vi "Get Session Info - 1Pin MSess .vi"(8 "error in":errorcluster, 10 "pin or relay name":string, 11 "session reservation in":refnum<class "Session Reservation.lvclass">) -> (0 "error out":errorcluster, 2 "sessions info":T1[](array[typedef]), 3 "session reservation out":refnum<class "Session Reservation.lvclass">)   [LabVIEW 2020, in "MeasurementLink Session Management.lvlib" / "Session Reservation.lvclass"]
doc: "Gets the connection information for the given <b>pin type</b>, <b>pin or relay name</b>, <b>instrument</b>, and <b>site</b>.The <b>instrument</b> input must return a valid instrument_type_id from the <b>Get Instrument Type ID.vi</b> override. The <b>connection type</b> input should be a cluster with two elements. The first element is a <b>Connection.ctl</b> cluster. The second element is the type of the session."
uses:
  Session Reservation.lvclass
  Session Reservation.lvclass/Session Reservation.ctl
  MeasurementLink Session Management Client/RPC Messages/nidevice_grpc_Session.ctl
  MeasurementLink Session Management Client/MeasurementLink Session Management Client.lvlib
  MeasurementLink Session Management Client/RPC Messages/ni_measurementlink_sessionmanagement_v1_ChannelMapping.ctl
  MeasurementLink Session Management Client/RPC Messages/ni_measurementlink_sessionmanagement_v1_SessionInformation.ctl
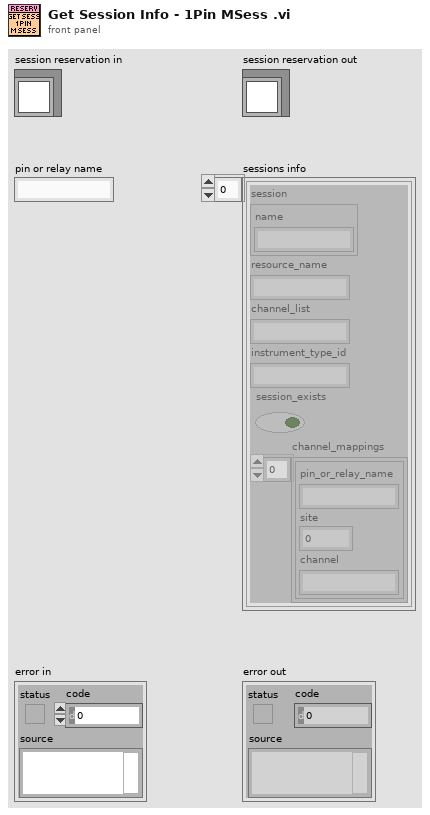
[diagram p1: front panel]
types:
  T1 = typedef "MeasurementLink Session Management Client.lvlib/ni_measurementlink_sessionmanagement_v1_SessionInformation.ctl" = cluster{"session":T2, "resource_name":string, "channel_list":string, "instrument_type_id":string, "session_exists":bool, "channel_mappings":T3[]}
  T2 = typedef "MeasurementLink Session Management Client.lvlib/nidevice_grpc_Session.ctl" = cluster{"name":string}
  T3 = typedef "MeasurementLink Session Management Client.lvlib/ni_measurementlink_sessionmanagement_v1_ChannelMapping.ctl" = cluster{"pin_or_relay_name":string, "site":i32, "channel":string}
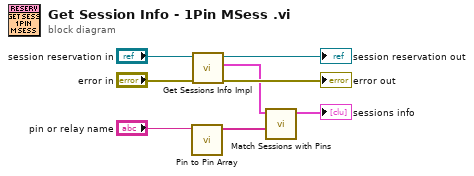
[diagram p0: block diagram]
diagram:
  n1 = call "Pin to Pin Array.vi"("pin or relay name"="pin or relay name") -> ("pin array"=w1:string[])  [unwired: 10 in]
  n2 = call "Get Sessions Info Impl.vi"("error in"="error in", "session reservation in"="session reservation in") -> ("error out"=→"error out":errorcluster, "sessions info"=w2:T1[], "session reservation out"=→"session reservation out":refnum<class "Session Reservation.lvclass">)  [unwired: 7 in]
  n3 = call "Match Sessions with Pins.vi"("pin array"=w1, "Sessions Info In"=w2) -> ("Sessions Info Out"=→"sessions info":T1[])  [unwired: 9 in]
